vi "CE14. Read_Voltage(subVI).vi"(8 "error in (no error)":errorcluster, 9 "milliseconds to wait(100)":u32=100, 11 "VISA resource name":refnum<visa-resource-name>) -> (0 "error out":errorcluster, 1 "data out":T1, 2 "read buffer":string, 3 "VISA resource name out":refnum<visa-resource-name>)   [LabVIEW 2018, in "CE14_eMIC.lvlib"]
uses:
  CE14_eMIC.lvlib
  type defs/CE14.data.ctl
  <vilib>/Instr/_visa.llb/VISA Flush IO Buffer Mask.ctl
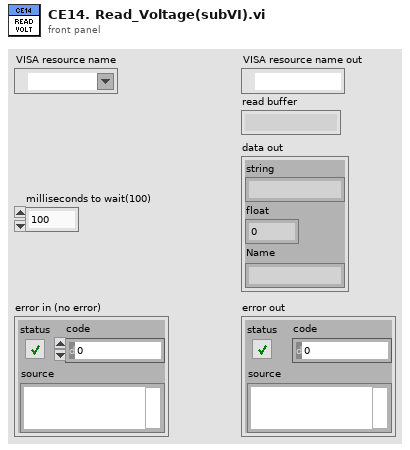
[diagram p1: front panel]
types:
  T1 = typedef "CE14_eMIC.lvlib/CE14.data.ctl" = cluster{"string":string, "float":dbl, "Name":string}
  T2 = typedef "VISA Flush IO Buffer Mask.ctl" = u16
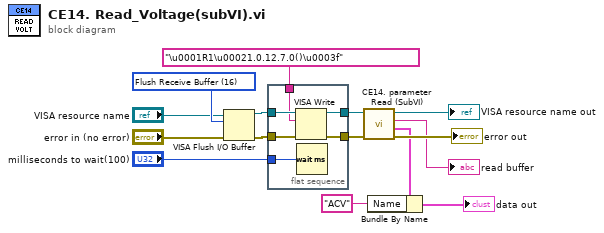
[diagram p0: block diagram]
diagram:
  w11 = T2 16 items=["Flush Receive Buffer"=16, "Write Transmit Buffer to Device"=32, "Flush Receive Buffer (No I/O)"=64, "Flush Transmit Buffer"=128] ("Mask")
  n1 = VISA Flush I/O Buffer(VISA resource name="VISA resource name", mask (16)=w11, error in (no error)="error in (no error)") -> (VISA resource name out=w12:refnum<visa-resource-name>, error out=w13:errorcluster)
  n2 = flat-sequence {
    tunnel: w12 -> [w21]
    tunnel: w13 -> [w20]
    tunnel: [w19] -> w14
    tunnel: [w18] -> w15
    tunnel: "\u0001R1\u00021.0.12.7.0()\u0003f" -> [w17]
    tunnel: "milliseconds to wait(100)" -> [w16]
    frame #0 {
      n3 = VISA Write(VISA resource name=w21, write buffer=w17, error in (no error)=w20) -> (VISA resource name out=w18:refnum<visa-resource-name>, error out=w19:errorcluster)  [unwired: 1 out]
      n4 = Wait (ms)(milliseconds to wait=w16) -> ()  [unwired: 1 out]
    }
  }
  n5 = call "CE14. parameter Read (SubVI).vi"("error in (no error)"=w14, "VISA Refnum in"=w15) -> ("error out"=→"error out":errorcluster, "dataout"=w3:T1, "read buffer"=→"read buffer":string, "VISA Refnum out"=→"VISA resource name out":refnum<visa-resource-name>)  [unwired: 5 in, 1 out]
  n6 = Bundle By Name(cluster=w3, "Name"="ACV") -> (→"data out":T1)
